vi "Lab Panel V5.22.1.vi"() -> ()   [LabVIEW 2013] (continued)
                            n1106 = Bundle(cluster=w2132, "STATUS"=w2129) -> (w2130:T4)  [unwired: 2 in]
                            n1107 = local write "RESULT LAB01-1"(TRUE) -> ()
                            n1108 = local write "DISP LAB01-1"(w2130) -> ()
                          }
                        }
                      }
                      frame False {
                      }
                    }
                  }
                }
              }
              frame #1 {
                # "LAB01-2"
                n1109 = Less?(x=w2133, y=2) -> (x < y?=w2136:bool)
                n1110 = local read "DISP LAB01-2"() -> (w2138:T4)
                n1111 = Unbundle(w2138) -> ("STATUS"=w2139:string)  [unwired: 2 out]
                n1112 = Equal?(x=w2139, y="RUN") -> (x = y?=w2135:bool)
                n1113 = And(x=w2135, y=w2136) -> (x .and. y?=w2134:bool)
                n1114 = case shown="True" w2134 {
                  tunnel: w2138 -> [_ w2144]
                  tunnel: w2133 -> [_ w2148]
                  frame False {
                  }
                  frame True {
                    n1115 = local read "SET LAB01-2"() -> (w2150:T5)
                    n1116 = local read "TDMS LAB01-2"() -> (w2143:refnum<k34>)
                    n1117 = Unbundle(w2150) -> ("CYCLES"=w2141:dbl, "T-RISE mins"=w2147:dbl)  [unwired: 3 out]
                    n1118 = case shown="\"T-RISE TEST\"" w2148 {
                      tunnel: w2147 -> [_ _ w2157]
                      tunnel: [w2152 w2154 w2157] -> w2146
                      tunnel: w2141 -> [w2152 w2154 _]
                      tunnel: ["CHART PASS" "CYCLE PASS" "T-RISE PASS"] -> w2145
                      frame "CHART TEST", Default {
                      }
                      frame "CYCLE TEST" {
                      }
                      frame "T-RISE TEST" {
                      }
                    }
                    n1119 = Unbundle(w2144) -> ("CYCLE"=w2149:dbl)  [unwired: 2 out]
                    n1120 = Increment(x=w2141) -> (x+1=w2142:dbl)
                    n1121 = Greater Or Equal?(x=w2149, y=w2142) -> (x >= y?=w2151:bool)
                    n1122 = case shown="True" w2151 {
                      tunnel: w2146 -> [w2161 _]
                      tunnel: w2145 -> [w2160 _]
                      tunnel: w2144 -> [w2159 _]
                      tunnel: w2143 -> [w2158 _]
                      frame True {
                        n1123 = stacked-sequence {
                          tunnel: w2161 -> [w2165 _]
                          tunnel: w2160 -> [w2163 w2169]
                          tunnel: w2159 -> [_ w2172]
                          tunnel: w2158 -> [w2162 _]
                          frame #0 {
                            n1124 = Build Array(w2163) -> (w2166:string[])
                            n1125 = Build Array(w2165) -> (w2164:dbl[])
                            n1126 = TDMS Write(0:w2162, 5:"TEST PASS", 7:w2166, 9:w2164) -> (15:w2168:errorcluster)  [unwired: 2 in, 3 out]
                            n1127 = local write "data file error"(w2168) -> ()
                          }
                          frame #1 {
                            n1128 = Bundle(cluster=w2172, "STATUS"=w2169) -> (w2170:T4)  [unwired: 2 in]
                            n1129 = local write "RESULT LAB01-2"(TRUE) -> ()
                            n1130 = local write "DISP LAB01-2"(w2170) -> ()
                          }
                        }
                      }
                      frame False {
                      }
                    }
                  }
                }
              }
              frame #2 {
                # "LAB02-1"
                n1131 = Less?(x=w2173, y=2) -> (x < y?=w2176:bool)
                n1132 = local read "DISP LAB02-1"() -> (w2178:T4)
                n1133 = Unbundle(w2178) -> ("STATUS"=w2179:string)  [unwired: 2 out]
                n1134 = Equal?(x=w2179, y="RUN") -> (x = y?=w2175:bool)
                n1135 = And(x=w2175, y=w2176) -> (x .and. y?=w2174:bool)
                n1136 = case shown="True" w2174 {
                  tunnel: w2178 -> [_ w2184]
                  tunnel: w2173 -> [_ w2188]
                  frame False {
                  }
                  frame True {
                    n1137 = local read "SET LAB02-1"() -> (w2190:T5)
                    n1138 = local read "TDMS LAB02-1"() -> (w2183:refnum<k34>)
                    n1139 = Unbundle(w2184) -> ("CYCLE"=w2189:dbl)  [unwired: 2 out]
                    n1140 = Unbundle(w2190) -> ("CYCLES"=w2181:dbl, "T-RISE mins"=w2187:dbl)  [unwired: 3 out]
                    n1141 = case shown="\"T-RISE TEST\"" w2188 {
                      tunnel: w2187 -> [_ _ w2197]
                      tunnel: [w2192 w2194 w2197] -> w2186
                      tunnel: w2181 -> [w2192 w2194 _]
                      tunnel: ["CHART PASS" "CYCLE PASS" "T-RISE PASS"] -> w2185
                      frame "CHART TEST", Default {
                      }
                      frame "CYCLE TEST" {
                      }
                      frame "T-RISE TEST" {
                      }
                    }
                    n1142 = Increment(x=w2181) -> (x+1=w2182:dbl)
                    n1143 = Greater Or Equal?(x=w2189, y=w2182) -> (x >= y?=w2191:bool)
                    n1144 = case shown="True" w2191 {
                      tunnel: w2186 -> [w2201 _]
                      tunnel: w2185 -> [w2200 _]
                      tunnel: w2184 -> [w2199 _]
                      tunnel: w2183 -> [w2198 _]
                      frame True {
                        n1145 = stacked-sequence {
                          tunnel: w2201 -> [w2205 _]
                          tunnel: w2200 -> [w2203 w2209]
                          tunnel: w2199 -> [_ w2212]
                          tunnel: w2198 -> [w2202 _]
                          frame #0 {
                            n1146 = Build Array(w2203) -> (w2206:string[])
                            n1147 = Build Array(w2205) -> (w2204:dbl[])
                            n1148 = TDMS Write(0:w2202, 5:"TEST PASS", 7:w2206, 9:w2204) -> (15:w2208:errorcluster)  [unwired: 2 in, 3 out]
                            n1149 = local write "data file error"(w2208) -> ()
                          }
                          frame #1 {
                            n1150 = Bundle(cluster=w2212, "STATUS"=w2209) -> (w2210:T4)  [unwired: 2 in]
                            n1151 = local write "RESULT LAB02-1"(TRUE) -> ()
                            n1152 = local write "DISP LAB02-1"(w2210) -> ()
                          }
                        }
                      }
                      frame False {
                      }
                    }
                  }
                }
              }
              frame #3 {
                # "LAB02-2"
                n1153 = Less?(x=w2213, y=2) -> (x < y?=w2216:bool)
                n1154 = local read "DISP LAB02-2"() -> (w2218:T4)
                n1155 = Unbundle(w2218) -> ("STATUS"=w2219:string)  [unwired: 2 out]
                n1156 = Equal?(x=w2219, y="RUN") -> (x = y?=w2215:bool)
                n1157 = And(x=w2215, y=w2216) -> (x .and. y?=w2214:bool)
                n1158 = case shown="True" w2214 {
                  tunnel: w2218 -> [_ w2224]
                  tunnel: w2213 -> [_ w2228]
                  frame False {
                  }
                  frame True {
                    n1159 = local read "SET LAB02-2"() -> (w2230:T5)
                    n1160 = local read "TDMS LAB02-2"() -> (w2223:refnum<k34>)
                    n1161 = Unbundle(w2224) -> ("CYCLE"=w2229:dbl)  [unwired: 2 out]
                    n1162 = Unbundle(w2230) -> ("CYCLES"=w2221:dbl, "T-RISE mins"=w2227:dbl)  [unwired: 3 out]
                    n1163 = case shown="\"T-RISE TEST\"" w2228 {
                      tunnel: w2227 -> [_ _ w2237]
                      tunnel: [w2232 w2234 w2237] -> w2226
                      tunnel: w2221 -> [w2232 w2234 _]
                      tunnel: ["CHART PASS" "CYCLE PASS" "T-RISE PASS"] -> w2225
                      frame "CHART TEST", Default {
                      }
                      frame "CYCLE TEST" {
                      }
                      frame "T-RISE TEST" {
                      }
                    }
                    n1164 = Increment(x=w2221) -> (x+1=w2222:dbl)
                    n1165 = Greater Or Equal?(x=w2229, y=w2222) -> (x >= y?=w2231:bool)
                    n1166 = case shown="True" w2231 {
                      tunnel: w2226 -> [w2241 _]
                      tunnel: w2225 -> [w2240 _]
                      tunnel: w2224 -> [w2239 _]
                      tunnel: w2223 -> [w2238 _]
                      frame True {
                        n1167 = stacked-sequence {
                          tunnel: w2241 -> [w2245 _]
                          tunnel: w2240 -> [w2243 w2249]
                          tunnel: w2239 -> [_ w2252]
                          tunnel: w2238 -> [w2242 _]
                          frame #0 {
                            n1168 = Build Array(w2243) -> (w2246:string[])
                            n1169 = Build Array(w2245) -> (w2244:dbl[])
                            n1170 = TDMS Write(0:w2242, 5:"TEST PASS", 7:w2246, 9:w2244) -> (15:w2248:errorcluster)  [unwired: 2 in, 3 out]
                            n1171 = local write "data file error"(w2248) -> ()
                          }
                          frame #1 {
                            n1172 = Bundle(cluster=w2252, "STATUS"=w2249) -> (w2250:T4)  [unwired: 2 in]
                            n1173 = local write "RESULT LAB02-2"(TRUE) -> ()
                            n1174 = local write "DISP LAB02-2"(w2250) -> ()
                          }
                        }
                      }
                      frame False {
                      }
                    }
                  }
                }
              }
              frame #4 {
                # "LAB03-1"
                n1175 = Less?(x=w2253, y=2) -> (x < y?=w2256:bool)
                n1176 = local read "DISP LAB03-1"() -> (w2258:T4)
                n1177 = Unbundle(w2258) -> ("STATUS"=w2259:string)  [unwired: 2 out]
                n1178 = Equal?(x=w2259, y="RUN") -> (x = y?=w2255:bool)
                n1179 = And(x=w2255, y=w2256) -> (x .and. y?=w2254:bool)
                n1180 = case shown="True" w2254 {
                  tunnel: w2258 -> [_ w2264]
                  tunnel: w2253 -> [_ w2268]
                  frame False {
                  }
                  frame True {
                    n1181 = local read "SET LAB03-1"() -> (w2270:T5)
                    n1182 = local read "TDMS LAB03-1"() -> (w2263:refnum<k34>)
                    n1183 = Unbundle(w2264) -> ("CYCLE"=w2269:dbl)  [unwired: 2 out]
                    n1184 = Unbundle(w2270) -> ("CYCLES"=w2261:dbl, "T-RISE mins"=w2267:dbl)  [unwired: 3 out]
                    n1185 = case shown="\"T-RISE TEST\"" w2268 {
                      tunnel: w2267 -> [_ _ w2277]
                      tunnel: [w2272 w2274 w2277] -> w2266
                      tunnel: w2261 -> [w2272 w2274 _]
                      tunnel: ["CHART PASS" "CYCLE PASS" "T-RISE PASS"] -> w2265
                      frame "CHART TEST", Default {
                      }
                      frame "CYCLE TEST" {
                      }
                      frame "T-RISE TEST" {
                      }
                    }
                    n1186 = Increment(x=w2261) -> (x+1=w2262:dbl)
                    n1187 = Greater Or Equal?(x=w2269, y=w2262) -> (x >= y?=w2271:bool)
                    n1188 = case shown="True" w2271 {
                      tunnel: w2266 -> [w2281 _]
                      tunnel: w2265 -> [w2280 _]
                      tunnel: w2264 -> [w2279 _]
                      tunnel: w2263 -> [w2278 _]
                      frame True {
                        n1189 = stacked-sequence {
                          tunnel: w2281 -> [w2285 _]
                          tunnel: w2280 -> [w2283 w2289]
                          tunnel: w2279 -> [_ w2292]
                          tunnel: w2278 -> [w2282 _]
                          frame #0 {
                            n1190 = Build Array(w2283) -> (w2286:string[])
                            n1191 = Build Array(w2285) -> (w2284:dbl[])
                            n1192 = TDMS Write(0:w2282, 5:"TEST PASS", 7:w2286, 9:w2284) -> (15:w2288:errorcluster)  [unwired: 2 in, 3 out]
                            n1193 = local write "data file error"(w2288) -> ()
                          }
                          frame #1 {
                            n1194 = Bundle(cluster=w2292, "STATUS"=w2289) -> (w2290:T4)  [unwired: 2 in]
                            n1195 = local write "RESULT LAB03-1"(TRUE) -> ()
                            n1196 = local write "DISP LAB03-1"(w2290) -> ()
                          }
                        }
                      }
                      frame False {
                      }
                    }
                  }
                }
              }
              frame #5 {
                # "LAB03-2"
                n1197 = Less?(x=w2293, y=2) -> (x < y?=w2296:bool)
                n1198 = local read "DISP LAB03-2"() -> (w2298:T4)
                n1199 = Unbundle(w2298) -> ("STATUS"=w2299:string)  [unwired: 2 out]
                n1200 = Equal?(x=w2299, y="RUN") -> (x = y?=w2295:bool)
                n1201 = And(x=w2295, y=w2296) -> (x .and. y?=w2294:bool)
                n1202 = case shown="True" w2294 {
                  tunnel: w2298 -> [_ w2304]
                  tunnel: w2293 -> [_ w2308]
                  frame False {
                  }
                  frame True {
                    n1203 = local read "SET LAB03-2"() -> (w2310:T5)
                    n1204 = local read "TDMS LAB03-2"() -> (w2303:refnum<k34>)
                    n1205 = Unbundle(w2304) -> ("CYCLE"=w2309:dbl)  [unwired: 2 out]
                    n1206 = Unbundle(w2310) -> ("CYCLES"=w2301:dbl, "T-RISE mins"=w2307:dbl)  [unwired: 3 out]
                    n1207 = case shown="\"T-RISE TEST\"" w2308 {
                      tunnel: w2307 -> [_ _ w2317]
                      tunnel: [w2312 w2314 w2317] -> w2306
                      tunnel: w2301 -> [w2312 w2314 _]
                      tunnel: ["CHART PASS" "CYCLE PASS" "T-RISE PASS"] -> w2305
                      frame "CHART TEST", Default {
                      }
                      frame "CYCLE TEST" {
                      }
                      frame "T-RISE TEST" {
                      }
                    }
                    n1208 = Increment(x=w2301) -> (x+1=w2302:dbl)
                    n1209 = Greater Or Equal?(x=w2309, y=w2302) -> (x >= y?=w2311:bool)
                    n1210 = case shown="True" w2311 {
                      tunnel: w2306 -> [w2321 _]
                      tunnel: w2305 -> [w2320 _]
                      tunnel: w2304 -> [w2319 _]
                      tunnel: w2303 -> [w2318 _]
                      frame True {
                        n1211 = stacked-sequence {
                          tunnel: w2321 -> [w2325 _]
                          tunnel: w2320 -> [w2323 w2329]
                          tunnel: w2319 -> [_ w2332]
                          tunnel: w2318 -> [w2322 _]
                          frame #0 {
                            n1212 = Build Array(w2323) -> (w2326:string[])
                            n1213 = Build Array(w2325) -> (w2324:dbl[])
                            n1214 = TDMS Write(0:w2322, 5:"TEST PASS", 7:w2326, 9:w2324) -> (15:w2328:errorcluster)  [unwired: 2 in, 3 out]
                            n1215 = local write "data file error"(w2328) -> ()
                          }
                          frame #1 {
                            n1216 = Bundle(cluster=w2332, "STATUS"=w2329) -> (w2330:T4)  [unwired: 2 in]
                            n1217 = local write "RESULT LAB03-2"(TRUE) -> ()
                            n1218 = local write "DISP LAB03-2"(w2330) -> ()
                          }
                        }
                      }
                      frame False {
                      }
                    }
                  }
                }
              }
              frame #6 {
                # "LAB04-1"
                n1219 = Less?(x=w2333, y=2) -> (x < y?=w2336:bool)
                n1220 = local read "DISP LAB04-1"() -> (w2338:T4)
                n1221 = Unbundle(w2338) -> ("STATUS"=w2339:string)  [unwired: 2 out]
                n1222 = Equal?(x=w2339, y="RUN") -> (x = y?=w2335:bool)
                n1223 = And(x=w2335, y=w2336) -> (x .and. y?=w2334:bool)
                n1224 = case shown="True" w2334 {
                  tunnel: w2338 -> [_ w2344]
                  tunnel: w2333 -> [_ w2348]
                  frame False {
                  }
                  frame True {
                    n1225 = local read "SET LAB04-1"() -> (w2350:T5)
                    n1226 = local read "TDMS LAB04-1"() -> (w2343:refnum<k34>)
                    n1227 = Unbundle(w2344) -> ("CYCLE"=w2349:dbl)  [unwired: 2 out]
                    n1228 = Unbundle(w2350) -> ("CYCLES"=w2341:dbl, "T-RISE mins"=w2347:dbl)  [unwired: 3 out]
                    n1229 = case shown="\"T-RISE TEST\"" w2348 {
                      tunnel: w2347 -> [_ _ w2357]
                      tunnel: [w2352 w2354 w2357] -> w2346
                      tunnel: w2341 -> [w2352 w2354 _]
                      tunnel: ["CHART PASS" "CYCLE PASS" "T-RISE PASS"] -> w2345
                      frame "CHART TEST", Default {
                      }
                      frame "CYCLE TEST" {
                      }
                      frame "T-RISE TEST" {
                      }
                    }
                    n1230 = Increment(x=w2341) -> (x+1=w2342:dbl)
                    n1231 = Greater Or Equal?(x=w2349, y=w2342) -> (x >= y?=w2351:bool)
                    n1232 = case shown="True" w2351 {
                      tunnel: w2346 -> [w2361 _]
                      tunnel: w2345 -> [w2360 _]
                      tunnel: w2344 -> [w2359 _]
                      tunnel: w2343 -> [w2358 _]
                      frame True {
                        n1233 = stacked-sequence {
                          tunnel: w2361 -> [w2365 _]
                          tunnel: w2360 -> [w2363 w2369]
                          tunnel: w2359 -> [_ w2372]
                          tunnel: w2358 -> [w2362 _]
                          frame #0 {
                            n1234 = Build Array(w2363) -> (w2366:string[])
                            n1235 = Build Array(w2365) -> (w2364:dbl[])
                            n1236 = TDMS Write(0:w2362, 5:"TEST PASS", 7:w2366, 9:w2364) -> (15:w2368:errorcluster)  [unwired: 2 in, 3 out]
                            n1237 = local write "data file error"(w2368) -> ()
                          }
                          frame #1 {
                            n1238 = Bundle(cluster=w2372, "STATUS"=w2369) -> (w2370:T4)  [unwired: 2 in]
                            n1239 = local write "RESULT LAB04-1"(TRUE) -> ()
                            n1240 = local write "DISP LAB04-1"(w2370) -> ()
                          }
                        }
                      }
                      frame False {
                      }
                    }
                  }
                }
              }
              frame #7 {
                # "LAB04-2"
                n1241 = Less?(x=w2373, y=2) -> (x < y?=w2376:bool)
                n1242 = local read "DISP LAB04-2"() -> (w2378:T4)
                n1243 = Unbundle(w2378) -> ("STATUS"=w2379:string)  [unwired: 2 out]
                n1244 = Equal?(x=w2379, y="RUN") -> (x = y?=w2375:bool)
                n1245 = And(x=w2375, y=w2376) -> (x .and. y?=w2374:bool)
                n1246 = case shown="True" w2374 {
                  tunnel: w2378 -> [_ w2384]
                  tunnel: w2373 -> [_ w2388]
                  frame False {
                  }
                  frame True {
                    n1247 = local read "SET LAB04-2"() -> (w2390:T5)
                    n1248 = local read "TDMS LAB04-2"() -> (w2383:refnum<k34>)
                    n1249 = Unbundle(w2384) -> ("CYCLE"=w2389:dbl)  [unwired: 2 out]
                    n1250 = Unbundle(w2390) -> ("CYCLES"=w2381:dbl, "T-RISE mins"=w2387:dbl)  [unwired: 3 out]
                    n1251 = case shown="\"T-RISE TEST\"" w2388 {
                      tunnel: w2387 -> [_ _ w2397]
                      tunnel: [w2392 w2394 w2397] -> w2386
                      tunnel: w2381 -> [w2392 w2394 _]
                      tunnel: ["CHART PASS" "CYCLE PASS" "T-RISE PASS"] -> w2385
                      frame "CHART TEST", Default {
                      }
                      frame "CYCLE TEST" {
                      }
                      frame "T-RISE TEST" {
                      }
                    }
                    n1252 = Increment(x=w2381) -> (x+1=w2382:dbl)
                    n1253 = Greater Or Equal?(x=w2389, y=w2382) -> (x >= y?=w2391:bool)
                    n1254 = case shown="True" w2391 {
                      tunnel: w2386 -> [w2401 _]
                      tunnel: w2385 -> [w2400 _]
                      tunnel: w2384 -> [w2399 _]
                      tunnel: w2383 -> [w2398 _]
                      frame True {
                        n1255 = stacked-sequence {
                          tunnel: w2401 -> [w2405 _]
                          tunnel: w2400 -> [w2403 w2409]
                          tunnel: w2399 -> [_ w2412]
                          tunnel: w2398 -> [w2402 _]
                          frame #0 {
                            n1256 = Build Array(w2403) -> (w2406:string[])
                            n1257 = Build Array(w2405) -> (w2404:dbl[])
                            n1258 = TDMS Write(0:w2402, 5:"TEST PASS", 7:w2406, 9:w2404) -> (15:w2408:errorcluster)  [unwired: 2 in, 3 out]
                            n1259 = local write "data file error"(w2408) -> ()
                          }
                          frame #1 {
                            n1260 = Bundle(cluster=w2412, "STATUS"=w2409) -> (w2410:T4)  [unwired: 2 in]
                            n1261 = local write "RESULT LAB04-2"(TRUE) -> ()
                            n1262 = local write "DISP LAB04-2"(w2410) -> ()
                          }
                        }
                      }
                      frame False {
                      }
                    }
                  }
                }
              }
              frame #8 {
                # "LAB05-1"
                n1263 = Less?(x=w2413, y=2) -> (x < y?=w2416:bool)
                n1264 = local read "DISP LAB05-1"() -> (w2418:T4)
                n1265 = Unbundle(w2418) -> ("STATUS"=w2419:string)  [unwired: 2 out]
                n1266 = Equal?(x=w2419, y="RUN") -> (x = y?=w2415:bool)
                n1267 = And(x=w2415, y=w2416) -> (x .and. y?=w2414:bool)
                n1268 = case shown="True" w2414 {
                  tunnel: w2418 -> [_ w2424]
                  tunnel: w2413 -> [_ w2428]
                  frame False {
                  }
                  frame True {
                    n1269 = local read "SET LAB05-1"() -> (w2430:T5)
                    n1270 = local read "TDMS LAB05-1"() -> (w2423:refnum<k34>)
                    n1271 = Unbundle(w2424) -> ("CYCLE"=w2429:dbl)  [unwired: 2 out]
                    n1272 = Unbundle(w2430) -> ("CYCLES"=w2421:dbl, "T-RISE mins"=w2427:dbl)  [unwired: 3 out]
                    n1273 = case shown="\"T-RISE TEST\"" w2428 {
                      tunnel: w2427 -> [_ _ w2437]
                      tunnel: [w2432 w2434 w2437] -> w2426
                      tunnel: w2421 -> [w2432 w2434 _]
                      tunnel: ["CHART PASS" "CYCLE PASS" "T-RISE PASS"] -> w2425
                      frame "CHART TEST", Default {
                      }
                      frame "CYCLE TEST" {
                      }
                      frame "T-RISE TEST" {
                      }
                    }
                    n1274 = Increment(x=w2421) -> (x+1=w2422:dbl)
                    n1275 = Greater Or Equal?(x=w2429, y=w2422) -> (x >= y?=w2431:bool)
                    n1276 = case shown="True" w2431 {
                      tunnel: w2426 -> [w2441 _]
                      tunnel: w2425 -> [w2440 _]
                      tunnel: w2424 -> [w2439 _]
                      tunnel: w2423 -> [w2438 _]
                      frame True {
                        n1277 = stacked-sequence {
                          tunnel: w2441 -> [w2445 _]
                          tunnel: w2440 -> [w2443 w2449]
                          tunnel: w2439 -> [_ w2452]
                          tunnel: w2438 -> [w2442 _]
                          frame #0 {
                            n1278 = Build Array(w2443) -> (w2446:string[])
                            n1279 = Build Array(w2445) -> (w2444:dbl[])
                            n1280 = TDMS Write(0:w2442, 5:"TEST PASS", 7:w2446, 9:w2444) -> (15:w2448:errorcluster)  [unwired: 2 in, 3 out]
                            n1281 = local write "data file error"(w2448) -> ()
                          }
                          frame #1 {
                            n1282 = Bundle(cluster=w2452, "STATUS"=w2449) -> (w2450:T4)  [unwired: 2 in]
                            n1283 = local write "RESULT LAB05-1"(TRUE) -> ()
                            n1284 = local write "DISP LAB05-1"(w2450) -> ()
                          }
                        }
                      }
                      frame False {
                      }
                    }
                  }
                }
              }
              frame #9 {
                # "LAB05-2"
                n1285 = Less?(x=w2453, y=2) -> (x < y?=w2456:bool)
                n1286 = local read "DISP LAB05-2"() -> (w2458:T4)
                n1287 = Unbundle(w2458) -> ("STATUS"=w2459:string)  [unwired: 2 out]
                n1288 = Equal?(x=w2459, y="RUN") -> (x = y?=w2455:bool)
                n1289 = And(x=w2455, y=w2456) -> (x .and. y?=w2454:bool)
                n1290 = case shown="True" w2454 {
                  tunnel: w2458 -> [_ w2464]
                  tunnel: w2453 -> [_ w2468]
                  frame False {
                  }
                  frame True {
                    n1291 = local read "SET LAB05-2"() -> (w2470:T5)
                    n1292 = local read "TDMS LAB05-2"() -> (w2463:refnum<k34>)
                    n1293 = Unbundle(w2464) -> ("CYCLE"=w2469:dbl)  [unwired: 2 out]
                    n1294 = Unbundle(w2470) -> ("CYCLES"=w2461:dbl, "T-RISE mins"=w2467:dbl)  [unwired: 3 out]
                    n1295 = case shown="\"T-RISE TEST\"" w2468 {
                      tunnel: w2467 -> [_ _ w2477]
                      tunnel: [w2472 w2474 w2477] -> w2466
                      tunnel: w2461 -> [w2472 w2474 _]
                      tunnel: ["CHART PASS" "CYCLE PASS" "T-RISE PASS"] -> w2465
                      frame "CHART TEST", Default {
                      }
                      frame "CYCLE TEST" {
                      }
                      frame "T-RISE TEST" {
                      }
                    }
                    n1296 = Increment(x=w2461) -> (x+1=w2462:dbl)
                    n1297 = Greater Or Equal?(x=w2469, y=w2462) -> (x >= y?=w2471:bool)
                    n1298 = case shown="True" w2471 {
                      tunnel: w2466 -> [w2481 _]
                      tunnel: w2465 -> [w2480 _]
                      tunnel: w2464 -> [w2479 _]
                      tunnel: w2463 -> [w2478 _]
                      frame True {
                        n1299 = stacked-sequence {
                          tunnel: w2481 -> [w2485 _]
                          tunnel: w2480 -> [w2483 w2489]
                          tunnel: w2479 -> [_ w2492]
                          tunnel: w2478 -> [w2482 _]
                          frame #0 {
                            n1300 = Build Array(w2483) -> (w2486:string[])
                            n1301 = Build Array(w2485) -> (w2484:dbl[])
                            n1302 = TDMS Write(0:w2482, 5:"TEST PASS", 7:w2486, 9:w2484) -> (15:w2488:errorcluster)  [unwired: 2 in, 3 out]
                            n1303 = local write "data file error"(w2488) -> ()
                          }
                          frame #1 {
                            n1304 = Bundle(cluster=w2492, "STATUS"=w2489) -> (w2490:T4)  [unwired: 2 in]
                            n1305 = local write "RESULT LAB05-2"(TRUE) -> ()
                            n1306 = local write "DISP LAB05-2"(w2490) -> ()
                          }
                        }
                      }
                      frame False {
                      }
                    }
                  }
                }
              }
            }
          }
          frame #5 {
            # "check if test cycles reached for temperature rise test"
            n1307 = stacked-sequence {
              tunnel: w2522 -> [_ _ _ _ _ _ _ _ _ _]
              tunnel: w2521 -> [_ _ _ _ _ _ _ _ _ _]
              tunnel: w2520 -> [_ _ _ _ _ _ _ _ _ _]
              tunnel: w2519 -> [_ _ _ _ _ _ _ _ _ _]
              tunnel: w2518 -> [_ _ _ _ _ _ _ _ _ _]
              tunnel: w2517 -> [_ _ _ _ _ _ _ _ _ _]
              tunnel: w2516 -> [_ _ _ _ _ _ _ _ _ _]
              tunnel: w2515 -> [_ _ _ _ _ _ _ _ _ _]
              tunnel: w2514 -> [_ _ _ _ _ _ _ _ _ _]
              tunnel: w2513 -> [_ _ _ _ _ _ _ _ _ _]
              tunnel: w2512 -> [w2528 _ _ _ _ _ _ _ _ _]
              tunnel: w2502 -> [w2523 _ _ _ _ _ _ _ _ _]
              tunnel: w2511 -> [_ w2554 _ _ _ _ _ _ _ _]
              tunnel: w2510 -> [_ _ w2584 _ _ _ _ _ _ _]
              tunnel: w2509 -> [_ _ _ w2614 _ _ _ _ _ _]
              tunnel: w2508 -> [_ _ _ _ w2644 _ _ _ _ _]
              tunnel: w2507 -> [_ _ _ _ _ w2674 _ _ _ _]
              tunnel: w2506 -> [_ _ _ _ _ _ w2704 _ _ _]
              tunnel: w2505 -> [_ _ _ _ _ _ _ w2734 _ _]
              tunnel: w2504 -> [_ _ _ _ _ _ _ _ w2764 _]
              tunnel: w2503 -> [_ _ _ _ _ _ _ _ _ w2794]
              tunnel: w2501 -> [_ w2553 _ _ _ _ _ _ _ _]
              tunnel: w2500 -> [_ _ w2583 _ _ _ _ _ _ _]
              tunnel: w2499 -> [_ _ _ w2613 _ _ _ _ _ _]
              tunnel: w2498 -> [_ _ _ _ w2643 _ _ _ _ _]
              tunnel: w2497 -> [_ _ _ _ _ w2673 _ _ _ _]
              tunnel: w2496 -> [_ _ _ _ _ _ w2703 _ _ _]
              tunnel: w2495 -> [_ _ _ _ _ _ _ w2733 _ _]
              tunnel: w2494 -> [_ _ _ _ _ _ _ _ w2763 _]
              tunnel: w2493 -> [_ _ _ _ _ _ _ _ _ w2793]
              frame #0 {
                # "LAB01-1"
                n1308 = Equal?(x=w2528, y=2) -> (x = y?=w2526:bool)
                n1309 = local read "DISP LAB01-1"() -> (w2529:T4)
                n1310 = Unbundle(w2529) -> ("STATUS"=w2530:string)  [unwired: 2 out]
                n1311 = Equal?(x=w2530, y="RUN") -> (x = y?=w2525:bool)
                n1312 = And(x=w2525, y=w2526) -> (x .and. y?=w2524:bool)
                n1313 = case shown="True" w2524 {
                  tunnel: w2529 -> [_ w2533]
                  tunnel: w2523 -> [_ w2536]
                  frame False {
                  }
                  frame True {
                    n1314 = local read "SET LAB01-1"() -> (w2535:T5)
                    n1315 = local read "TDMS LAB01-1"() -> (w2532:refnum<k34>)
                    n1316 = Unbundle(w2533) -> ("CYCLE"=w2537:dbl)  [unwired: 2 out]
                    n1317 = Unbundle(w2535) -> ("T-RISE mins"=w2534:dbl)  [unwired: 4 out]
                    n1318 = Greater Or Equal?(x=w2537, y=w2536) -> (x >= y?=w2538:bool)
                    n1319 = case shown="True" w2538 {
                      tunnel: w2534 -> [w2541 _]
                      tunnel: w2533 -> [w2540 _]
                      tunnel: w2532 -> [w2539 _]
                      frame True {
                        n1320 = stacked-sequence {
                          tunnel: w2541 -> [w2544 _]
                          tunnel: w2540 -> [_ w2549]
                          tunnel: w2539 -> [w2542 _]
                          frame #0 {
                            n1321 = Build Array("T-RISE") -> (w2546:string[])
                            n1322 = Build Array(w2544) -> (w2545:dbl[])
                            n1323 = TDMS Write(0:w2542, 5:"TEST PASS", 7:w2546, 9:w2545) -> (15:w2548:errorcluster)  [unwired: 2 in, 3 out]
                            n1324 = local write "data file error"(w2548) -> ()
                          }
                          frame #1 {
                            n1325 = Bundle(cluster=w2549, "STATUS"="T-RISE PASS") -> (w2551:T4)  [unwired: 2 in]
                            n1326 = local write "RESULT LAB01-1"(TRUE) -> ()
                            n1327 = local write "DISP LAB01-1"(w2551) -> ()
                          }
                        }
                      }
                      frame False {
                      }
                    }
                  }
                }
              }
              frame #1 {
                # "LAB01-2"
                n1328 = Equal?(x=w2554, y=2) -> (x = y?=w2557:bool)
                n1329 = local read "DISP LAB01-2"() -> (w2559:T4)
                n1330 = Unbundle(w2559) -> ("STATUS"=w2560:string)  [unwired: 2 out]
                n1331 = Equal?(x=w2560, y="RUN") -> (x = y?=w2556:bool)
                n1332 = And(x=w2556, y=w2557) -> (x .and. y?=w2555:bool)
                n1333 = case shown="True" w2555 {
                  tunnel: w2559 -> [_ w2563]
                  tunnel: w2553 -> [_ w2566]
                  frame False {
                  }
                  frame True {
                    n1334 = local read "SET LAB01-2"() -> (w2565:T5)
                    n1335 = local read "TDMS LAB01-2"() -> (w2562:refnum<k34>)
                    n1336 = Unbundle(w2563) -> ("CYCLE"=w2567:dbl)  [unwired: 2 out]
                    n1337 = Unbundle(w2565) -> ("T-RISE mins"=w2564:dbl)  [unwired: 4 out]
                    n1338 = Greater Or Equal?(x=w2567, y=w2566) -> (x >= y?=w2568:bool)
                    n1339 = case shown="True" w2568 {
                      tunnel: w2564 -> [w2571 _]
                      tunnel: w2563 -> [w2570 _]
                      tunnel: w2562 -> [w2569 _]
                      frame True {
                        n1340 = stacked-sequence {
                          tunnel: w2571 -> [w2574 _]
                          tunnel: w2570 -> [_ w2579]
                          tunnel: w2569 -> [w2572 _]
                          frame #0 {
                            n1341 = Build Array("T-RISE") -> (w2576:string[])
                            n1342 = Build Array(w2574) -> (w2575:dbl[])
                            n1343 = TDMS Write(0:w2572, 5:"TEST PASS", 7:w2576, 9:w2575) -> (15:w2578:errorcluster)  [unwired: 2 in, 3 out]
                            n1344 = local write "data file error"(w2578) -> ()
                          }
                          frame #1 {
                            n1345 = Bundle(cluster=w2579, "STATUS"="T-RISE PASS") -> (w2581:T4)  [unwired: 2 in]
                            n1346 = local write "RESULT LAB01-2"(TRUE) -> ()
                            n1347 = local write "DISP LAB01-2"(w2581) -> ()
                          }
                        }
                      }
                      frame False {
                      }
                    }
                  }
                }
              }
              frame #2 {
                # "LAB02-1"
                n1348 = Equal?(x=w2584, y=2) -> (x = y?=w2587:bool)
                n1349 = local read "DISP LAB02-1"() -> (w2589:T4)
                n1350 = Unbundle(w2589) -> ("STATUS"=w2590:string)  [unwired: 2 out]
                n1351 = Equal?(x=w2590, y="RUN") -> (x = y?=w2586:bool)
                n1352 = And(x=w2586, y=w2587) -> (x .and. y?=w2585:bool)
                n1353 = case shown="True" w2585 {
                  tunnel: w2589 -> [_ w2593]
                  tunnel: w2583 -> [_ w2596]
                  frame False {
                  }
                  frame True {
                    n1354 = local read "SET LAB02-1"() -> (w2595:T5)
                    n1355 = local read "TDMS LAB02-1"() -> (w2592:refnum<k34>)
                    n1356 = Unbundle(w2593) -> ("CYCLE"=w2597:dbl)  [unwired: 2 out]
                    n1357 = Unbundle(w2595) -> ("T-RISE mins"=w2594:dbl)  [unwired: 4 out]
                    n1358 = Greater Or Equal?(x=w2597, y=w2596) -> (x >= y?=w2598:bool)
                    n1359 = case shown="True" w2598 {
                      tunnel: w2594 -> [w2601 _]
                      tunnel: w2593 -> [w2600 _]
                      tunnel: w2592 -> [w2599 _]
                      frame True {
                        n1360 = stacked-sequence {
                          tunnel: w2601 -> [w2604 _]
                          tunnel: w2600 -> [_ w2609]
                          tunnel: w2599 -> [w2602 _]
                          frame #0 {
                            n1361 = Build Array("T-RISE") -> (w2606:string[])
                            n1362 = Build Array(w2604) -> (w2605:dbl[])
                            n1363 = TDMS Write(0:w2602, 5:"TEST PASS", 7:w2606, 9:w2605) -> (15:w2608:errorcluster)  [unwired: 2 in, 3 out]
                            n1364 = local write "data file error"(w2608) -> ()
                          }
                          frame #1 {
                            n1365 = Bundle(cluster=w2609, "STATUS"="T-RISE PASS") -> (w2611:T4)  [unwired: 2 in]
                            n1366 = local write "RESULT LAB02-1"(TRUE) -> ()
                            n1367 = local write "DISP LAB02-1"(w2611) -> ()
                          }
                        }
                      }
                      frame False {
                      }
                    }
                  }
                }
              }
              frame #3 {
                # "LAB02-2"
                n1368 = Equal?(x=w2614, y=2) -> (x = y?=w2617:bool)
                n1369 = local read "DISP LAB02-2"() -> (w2619:T4)
                n1370 = Unbundle(w2619) -> ("STATUS"=w2620:string)  [unwired: 2 out]
                n1371 = Equal?(x=w2620, y="RUN") -> (x = y?=w2616:bool)
                n1372 = And(x=w2616, y=w2617) -> (x .and. y?=w2615:bool)
                n1373 = case shown="True" w2615 {
                  tunnel: w2619 -> [_ w2623]
                  tunnel: w2613 -> [_ w2626]
                  frame False {
                  }
                  frame True {
                    n1374 = local read "SET LAB02-2"() -> (w2625:T5)
                    n1375 = local read "TDMS LAB02-2"() -> (w2622:refnum<k34>)
                    n1376 = Unbundle(w2623) -> ("CYCLE"=w2627:dbl)  [unwired: 2 out]
                    n1377 = Unbundle(w2625) -> ("T-RISE mins"=w2624:dbl)  [unwired: 4 out]
                    n1378 = Greater Or Equal?(x=w2627, y=w2626) -> (x >= y?=w2628:bool)
                    n1379 = case shown="True" w2628 {
                      tunnel: w2624 -> [w2631 _]
                      tunnel: w2623 -> [w2630 _]
                      tunnel: w2622 -> [w2629 _]
                      frame True {
                        n1380 = stacked-sequence {
                          tunnel: w2631 -> [w2634 _]
                          tunnel: w2630 -> [_ w2639]
                          tunnel: w2629 -> [w2632 _]
                          frame #0 {
                            n1381 = Build Array("T-RISE") -> (w2636:string[])
                            n1382 = Build Array(w2634) -> (w2635:dbl[])
                            n1383 = TDMS Write(0:w2632, 5:"TEST PASS", 7:w2636, 9:w2635) -> (15:w2638:errorcluster)  [unwired: 2 in, 3 out]
                            n1384 = local write "data file error"(w2638) -> ()
                          }
                          frame #1 {
                            n1385 = Bundle(cluster=w2639, "STATUS"="T-RISE PASS") -> (w2641:T4)  [unwired: 2 in]
                            n1386 = local write "RESULT LAB02-2"(TRUE) -> ()
                            n1387 = local write "DISP LAB02-2"(w2641) -> ()
                          }
                        }
                      }
                      frame False {
                      }
                    }
                  }
                }
              }
              frame #4 {
                # "LAB03-1"
                n1388 = Equal?(x=w2644, y=2) -> (x = y?=w2647:bool)
                n1389 = local read "DISP LAB03-1"() -> (w2649:T4)
                n1390 = Unbundle(w2649) -> ("STATUS"=w2650:string)  [unwired: 2 out]
                n1391 = Equal?(x=w2650, y="RUN") -> (x = y?=w2646:bool)
                n1392 = And(x=w2646, y=w2647) -> (x .and. y?=w2645:bool)
                n1393 = case shown="True" w2645 {
                  tunnel: w2649 -> [_ w2653]
                  tunnel: w2643 -> [_ w2656]
                  frame False {
                  }
                  frame True {
                    n1394 = local read "SET LAB03-1"() -> (w2655:T5)
                    n1395 = local read "TDMS LAB03-1"() -> (w2652:refnum<k34>)
                    n1396 = Unbundle(w2653) -> ("CYCLE"=w2657:dbl)  [unwired: 2 out]
                    n1397 = Unbundle(w2655) -> ("T-RISE mins"=w2654:dbl)  [unwired: 4 out]
                    n1398 = Greater Or Equal?(x=w2657, y=w2656) -> (x >= y?=w2658:bool)
                    n1399 = case shown="True" w2658 {
                      tunnel: w2654 -> [w2661 _]
                      tunnel: w2653 -> [w2660 _]
                      tunnel: w2652 -> [w2659 _]
                      frame True {
                        n1400 = stacked-sequence {
                          tunnel: w2661 -> [w2664 _]
                          tunnel: w2660 -> [_ w2669]
                          tunnel: w2659 -> [w2662 _]
                          frame #0 {
                            n1401 = Build Array("T-RISE") -> (w2666:string[])
                            n1402 = Build Array(w2664) -> (w2665:dbl[])
                            n1403 = TDMS Write(0:w2662, 5:"TEST PASS", 7:w2666, 9:w2665) -> (15:w2668:errorcluster)  [unwired: 2 in, 3 out]
                            n1404 = local write "data file error"(w2668) -> ()
                          }
                          frame #1 {
                            n1405 = Bundle(cluster=w2669, "STATUS"="T-RISE PASS") -> (w2671:T4)  [unwired: 2 in]
                            n1406 = local write "RESULT LAB03-1"(TRUE) -> ()
                            n1407 = local write "DISP LAB03-1"(w2671) -> ()
                          }
                        }
                      }
                      frame False {
                      }
                    }
                  }
                }
              }
              frame #5 {
                # "LAB03-2"
                n1408 = Equal?(x=w2674, y=2) -> (x = y?=w2677:bool)
                n1409 = local read "DISP LAB03-2"() -> (w2679:T4)
                n1410 = Unbundle(w2679) -> ("STATUS"=w2680:string)  [unwired: 2 out]
                n1411 = Equal?(x=w2680, y="RUN") -> (x = y?=w2676:bool)
                n1412 = And(x=w2676, y=w2677) -> (x .and. y?=w2675:bool)
                n1413 = case shown="True" w2675 {
                  tunnel: w2679 -> [_ w2683]
                  tunnel: w2673 -> [_ w2686]
                  frame False {
                  }
                  frame True {
                    n1414 = local read "SET LAB03-2"() -> (w2685:T5)
                    n1415 = local read "TDMS LAB03-2"() -> (w2682:refnum<k34>)
                    n1416 = Unbundle(w2683) -> ("CYCLE"=w2687:dbl)  [unwired: 2 out]
                    n1417 = Unbundle(w2685) -> ("T-RISE mins"=w2684:dbl)  [unwired: 4 out]
                    n1418 = Greater Or Equal?(x=w2687, y=w2686) -> (x >= y?=w2688:bool)
                    n1419 = case shown="True" w2688 {
                      tunnel: w2684 -> [w2691 _]
                      tunnel: w2683 -> [w2690 _]
                      tunnel: w2682 -> [w2689 _]
                      frame True {
                        n1420 = stacked-sequence {
                          tunnel: w2691 -> [w2694 _]
                          tunnel: w2690 -> [_ w2699]
                          tunnel: w2689 -> [w2692 _]
                          frame #0 {
                            n1421 = Build Array("T-RISE") -> (w2696:string[])
                            n1422 = Build Array(w2694) -> (w2695:dbl[])
                            n1423 = TDMS Write(0:w2692, 5:"TEST PASS", 7:w2696, 9:w2695) -> (15:w2698:errorcluster)  [unwired: 2 in, 3 out]
                            n1424 = local write "data file error"(w2698) -> ()
                          }
                          frame #1 {
                            n1425 = Bundle(cluster=w2699, "STATUS"="T-RISE PASS") -> (w2701:T4)  [unwired: 2 in]
                            n1426 = local write "RESULT LAB03-2"(TRUE) -> ()
                            n1427 = local write "DISP LAB03-2"(w2701) -> ()
                          }
                        }
                      }
                      frame False {
                      }
                    }
                  }
                }
              }
              frame #6 {
                # "LAB04-1"
                n1428 = Equal?(x=w2704, y=2) -> (x = y?=w2707:bool)
                n1429 = local read "DISP LAB04-1"() -> (w2709:T4)
                n1430 = Unbundle(w2709) -> ("STATUS"=w2710:string)  [unwired: 2 out]
                n1431 = Equal?(x=w2710, y="RUN") -> (x = y?=w2706:bool)
                n1432 = And(x=w2706, y=w2707) -> (x .and. y?=w2705:bool)
                n1433 = case shown="True" w2705 {
                  tunnel: w2709 -> [_ w2713]
                  tunnel: w2703 -> [_ w2716]
                  frame False {
                  }
                  frame True {
                    n1434 = local read "SET LAB04-1"() -> (w2715:T5)
                    n1435 = local read "TDMS LAB04-1"() -> (w2712:refnum<k34>)
                    n1436 = Unbundle(w2713) -> ("CYCLE"=w2717:dbl)  [unwired: 2 out]
                    n1437 = Unbundle(w2715) -> ("T-RISE mins"=w2714:dbl)  [unwired: 4 out]
                    n1438 = Greater Or Equal?(x=w2717, y=w2716) -> (x >= y?=w2718:bool)
                    n1439 = case shown="True" w2718 {
                      tunnel: w2714 -> [w2721 _]
                      tunnel: w2713 -> [w2720 _]
                      tunnel: w2712 -> [w2719 _]
                      frame True {
                        n1440 = stacked-sequence {
                          tunnel: w2721 -> [w2724 _]
                          tunnel: w2720 -> [_ w2729]
                          tunnel: w2719 -> [w2722 _]
                          frame #0 {
                            n1441 = Build Array("T-RISE") -> (w2726:string[])
                            n1442 = Build Array(w2724) -> (w2725:dbl[])
                            n1443 = TDMS Write(0:w2722, 5:"TEST PASS", 7:w2726, 9:w2725) -> (15:w2728:errorcluster)  [unwired: 2 in, 3 out]
                            n1444 = local write "data file error"(w2728) -> ()
                          }
                          frame #1 {
                            n1445 = Bundle(cluster=w2729, "STATUS"="T-RISE PASS") -> (w2731:T4)  [unwired: 2 in]
                            n1446 = local write "RESULT LAB04-1"(TRUE) -> ()
                            n1447 = local write "DISP LAB04-1"(w2731) -> ()
                          }
                        }
                      }
                      frame False {
                      }
                    }
                  }
                }
              }
              frame #7 {
                # "LAB04-2"
                n1448 = Equal?(x=w2734, y=2) -> (x = y?=w2737:bool)
                n1449 = local read "DISP LAB04-2"() -> (w2739:T4)
                n1450 = Unbundle(w2739) -> ("STATUS"=w2740:string)  [unwired: 2 out]
                n1451 = Equal?(x=w2740, y="RUN") -> (x = y?=w2736:bool)
                n1452 = And(x=w2736, y=w2737) -> (x .and. y?=w2735:bool)
                n1453 = case shown="True" w2735 {
                  tunnel: w2739 -> [_ w2743]
                  tunnel: w2733 -> [_ w2746]
                  frame False {
                  }
                  frame True {
                    n1454 = local read "SET LAB04-2"() -> (w2745:T5)
                    n1455 = local read "TDMS LAB04-2"() -> (w2742:refnum<k34>)
                    n1456 = Unbundle(w2743) -> ("CYCLE"=w2747:dbl)  [unwired: 2 out]
                    n1457 = Unbundle(w2745) -> ("T-RISE mins"=w2744:dbl)  [unwired: 4 out]
                    n1458 = Greater Or Equal?(x=w2747, y=w2746) -> (x >= y?=w2748:bool)
                    n1459 = case shown="True" w2748 {
                      tunnel: w2744 -> [w2751 _]
                      tunnel: w2743 -> [w2750 _]
                      tunnel: w2742 -> [w2749 _]
                      frame True {
                        n1460 = stacked-sequence {
                          tunnel: w2751 -> [w2754 _]
                          tunnel: w2750 -> [_ w2759]
                          tunnel: w2749 -> [w2752 _]
                          frame #0 {
                            n1461 = Build Array("T-RISE") -> (w2756:string[])
                            n1462 = Build Array(w2754) -> (w2755:dbl[])
                            n1463 = TDMS Write(0:w2752, 5:"TEST PASS", 7:w2756, 9:w2755) -> (15:w2758:errorcluster)  [unwired: 2 in, 3 out]
                            n1464 = local write "data file error"(w2758) -> ()
                          }
                          frame #1 {
                            n1465 = Bundle(cluster=w2759, "STATUS"="T-RISE PASS") -> (w2761:T4)  [unwired: 2 in]
